vi "Programa_da_Aplicação_Hold_UP.vi"() -> ()   [LabVIEW 2019]
uses:
  Variaveis_Globais_CLP_Paralelo.vi
panel:
  in  "SPW-INV-001":bool
  in  "SPK-INV-001":bool
  in  "Condição_Hold_up_Vini":bool
  in  "Valores_Instrumentos":T1 {"DeltaP_K" format="%#_6e"; "DeltaP_W" format="%#_6e"; "Diâmetro Tubulação [m]" format="%#_6e"; "PC-TQ-TD" format="%#_6e"; "PC-TQ-TI" format="%#_6e"; "PC-TQ-GP" format="%#_6e"; "PC-TQ-PV" format="%#_6e"; "PC-TQ-SP" format="%#_6e"; "PC-TQ-OV" format="%#_6e"; "SPW-WR-VEL" format="%#_6e"; "SPK-WR-VEL" format="%#_6e"; "SKM-PC-TQ" format="%#_6e"; "SKM-FC-KF" format="%#_6e"; "SKM-FC-WF" format="%#_6e"; "SKM-FC-AR" format="%#_6e"; "SKM-TI-KF_COR" format="%#_6e"; "SKS-LC-K" format="%#_6e"; "SPK-RD-CRT" format="%#_6e"; "SPW-RD-CRT" format="%#_6e"; "SKM-FIC-AR_COR" format="%#_6e"; "SKM-FIC-KF_COR" format="%#_6e"; "SKM-AI-AR_COR" format="%#_6e"; "SKM-AI-KF_COR" format="%#_6e"; "SKM-TI-AR_COR" format="%#_6e"; "SKM-TI-KF" format="%#_6e"; "SPW-RD-VEL" format="%#_6e"; "SPK-RD-VEL" format="%#_6e"; "SKS-LC-W" format="%#_6e"; "SIT-PI-002" format="%#_6e"; "SKM-FI-WF" format="%#_6e"; "SKM-TI-WF" format="%#_6e"; "SKM-PI-BAR" format="%#_6e"; "SKM-PI-LAM" format="%#_6e"; "SMA-PI-LAM" format="%#_6e"; "SMA-TI-LAM" format="%#_6e"; "SKM-PI-TQ" format="%#_6e"; "SKM-TI-TQ" format="%#_6e"}
  in  "stop":bool
  in  "SPK-WR-VEL":dbl caption="SPK-WR-VEL [%]"
  in  "SPW-WR-VEL":dbl caption="SPW-WR-VEL [%]"
  in  "SKM-FC-TQ":dbl caption="SKM-FC-TQ [%]"
  in  "SKM-FC-AR":dbl caption="SKM-FC-AR [%]"
  in  "SKM-FC-WF":dbl caption="SKM-FC-WF [%]"
  in  "SKM-FC-KF":dbl caption="SKM-FC-KF [%]"
  in  "Variaveis_Aplicações":T2
  # "Controle de Valvulas"
  # "Controle de Bombas"
  # "Espaço Delimitado para criação do Painel Frontal \nque será utilizado nessa aplicação."
  # "SKID MEDI敲O - LEITURA"
  # "SKID MEDI敲O - ESCRITA"
  # "SKID BOMBA - ESCRITA"
  # "SKID BOMBA - LEITURA"
  # "SKID SEPARA敲O - LEITURA"
  # "SKID INJE敲O - LEITURA"
  # "SKID BOMBA"
  # "SKID DE MEDI敲O"
  # "SKID DE SEPARA敲O"
  # "SKID DE INJE敲O"
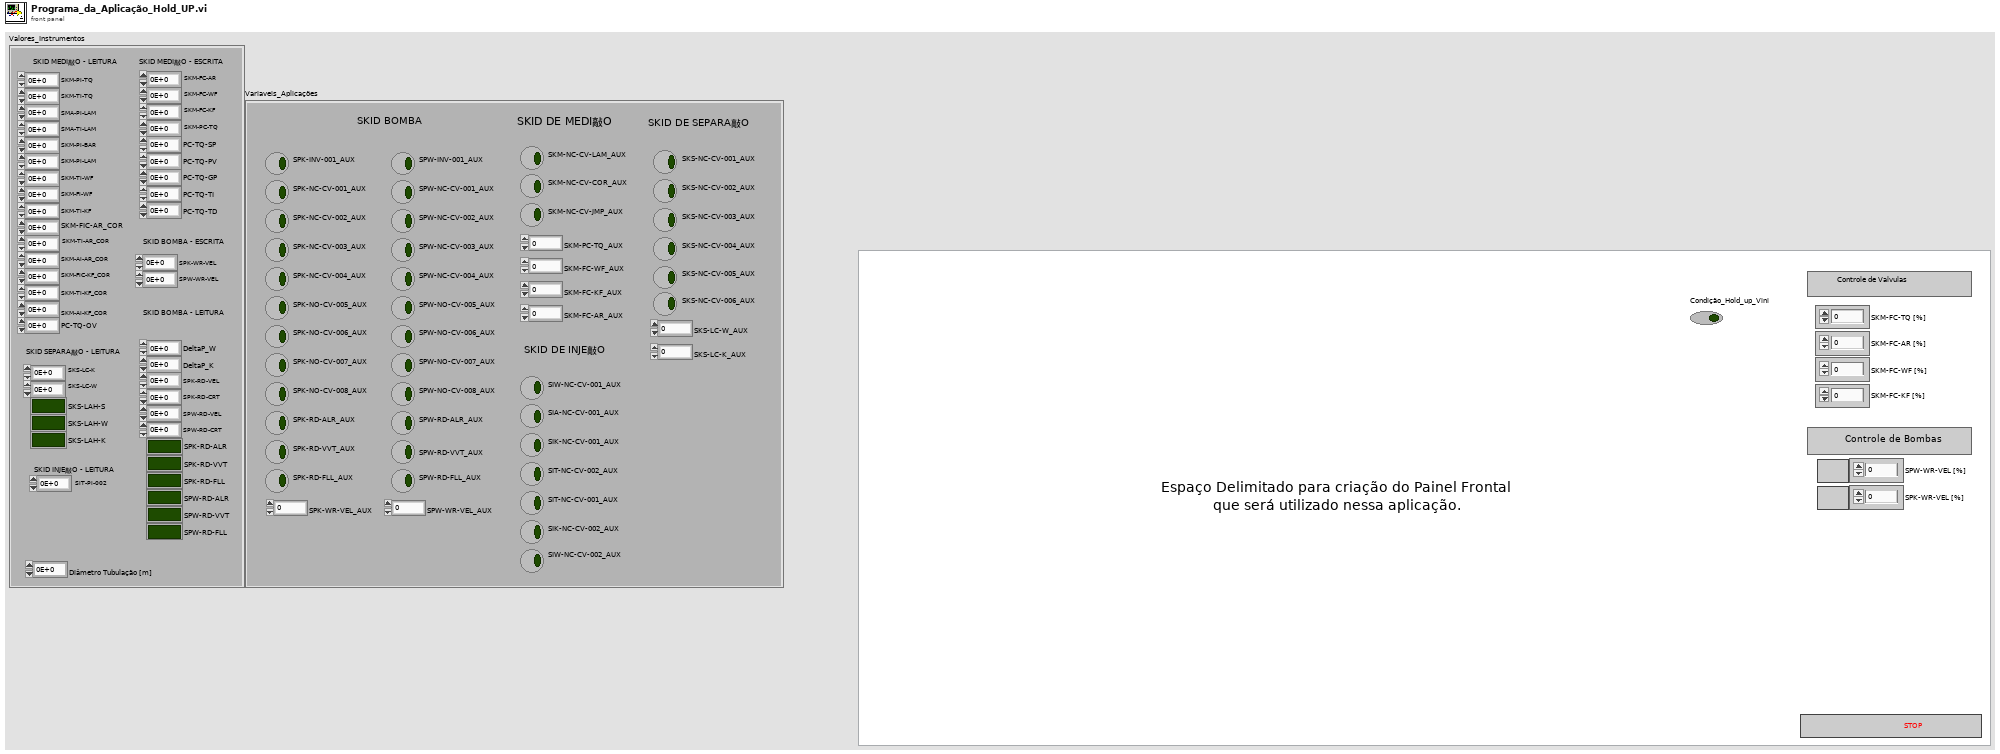
[diagram p1: front panel]
types:
  T1 = cluster{"SKM-TI-TQ":dbl, "SKM-PI-TQ":dbl, "SMA-TI-LAM":dbl, "SMA-PI-LAM":dbl, "SKM-PI-LAM":dbl, "SKM-PI-BAR":dbl, "SKM-TI-WF":dbl, "SKM-FI-WF":dbl, "SIT-PI-002":dbl, "SKS-LC-W":dbl, "SPK-RD-VEL":dbl, "SPW-RD-VEL":dbl, "SKM-TI-KF":dbl, "SKM-TI-AR_COR":dbl, "SKM-AI-KF_COR":dbl, "SKM-AI-AR_COR":dbl, "SKM-FIC-KF_COR":dbl, "SKM-FIC-AR_COR":dbl, "SPW-RD-CRT":dbl, "SPK-RD-CRT":dbl, "SKS-LC-K":dbl, "SKM-TI-KF_COR":dbl, "SKM-FC-AR":dbl, "SKM-FC-WF":dbl, "SKM-FC-KF":dbl, "SKM-PC-TQ":dbl, "SPK-WR-VEL":dbl, "SPW-WR-VEL":dbl, "SPK-RD-ALR":bool, "SPK-RD-VVT":bool, "SPK-RD-FLL":bool, "SPW-RD-ALR":bool, "SPW-RD-VVT":bool, "SPW-RD-FLL":bool, "PC-TQ-OV":dbl, "PC-TQ-SP":dbl, "PC-TQ-PV":dbl, "PC-TQ-GP":dbl, "PC-TQ-TI":dbl, "PC-TQ-TD":dbl, "SKS-LAH-S":bool, "SKS-LAH-W":bool, "SKS-LAH-K":bool, "Diâmetro Tubulação [m]":dbl, "DeltaP_W":dbl, "DeltaP_K":dbl}
  T2 = cluster{"SPK-NC-CV-001_AUX":bool, "SPK-NC-CV-002_AUX":bool, "SPK-NC-CV-003_AUX":bool, "SPK-NC-CV-004_AUX":bool, "SPK-NO-CV-005_AUX":bool, "SPK-NO-CV-006_AUX":bool, "SPK-NO-CV-007_AUX":bool, "SPK-NO-CV-008_AUX":bool, "SIW-NC-CV-001_AUX":bool, "SIA-NC-CV-001_AUX":bool, "SIK-NC-CV-001_AUX":bool, "SIT-NC-CV-002_AUX":bool, "SIT-NC-CV-001_AUX":bool, "SIK-NC-CV-002_AUX":bool, "SIW-NC-CV-002_AUX":bool, "SKS-NC-CV-001_AUX":bool, "SKS-NC-CV-002_AUX":bool, "SKS-NC-CV-003_AUX":bool, "SPK-INV-001_AUX":bool, "SPW-NC-CV-001_AUX":bool, "SPW-NC-CV-002_AUX":bool, "SPW-NC-CV-003_AUX":bool, "SPW-NC-CV-004_AUX":bool, "SPW-NO-CV-005_AUX":bool, "SPW-NO-CV-006_AUX":bool, "SPW-NO-CV-007_AUX":bool, "SPW-NO-CV-008_AUX":bool, "SPW-INV-001_AUX":bool, "SKM-NC-CV-LAM_AUX":bool, "SKM-NC-CV-COR_AUX":bool, "SKM-NC-CV-JMP_AUX":bool, "SKM-FC-AR_AUX":dbl, "SPK-RD-ALR_AUX":bool, "SPK-RD-VVT_AUX":bool, "SPK-RD-FLL_AUX":bool, "SPK-WR-VEL_AUX":dbl, "SPW-RD-ALR_AUX":bool, "SPW-RD-VVT_AUX ":bool, "SPW-RD-FLL_AUX ":bool, "SPW-WR-VEL_AUX ":dbl, "SKS-NC-CV-004_AUX":bool, "SKS-NC-CV-005_AUX":bool, "SKS-LC-W_AUX":dbl, "SKS-LC-K_AUX":dbl, "SKM-PC-TQ_AUX":dbl, "SKM-FC-WF_AUX":dbl, "SKM-FC-KF_AUX":dbl, "SKS-NC-CV-006_AUX":bool}
  T3 = enum8{"Enabled", "Disabled", "Disabled and Grayed Out"}
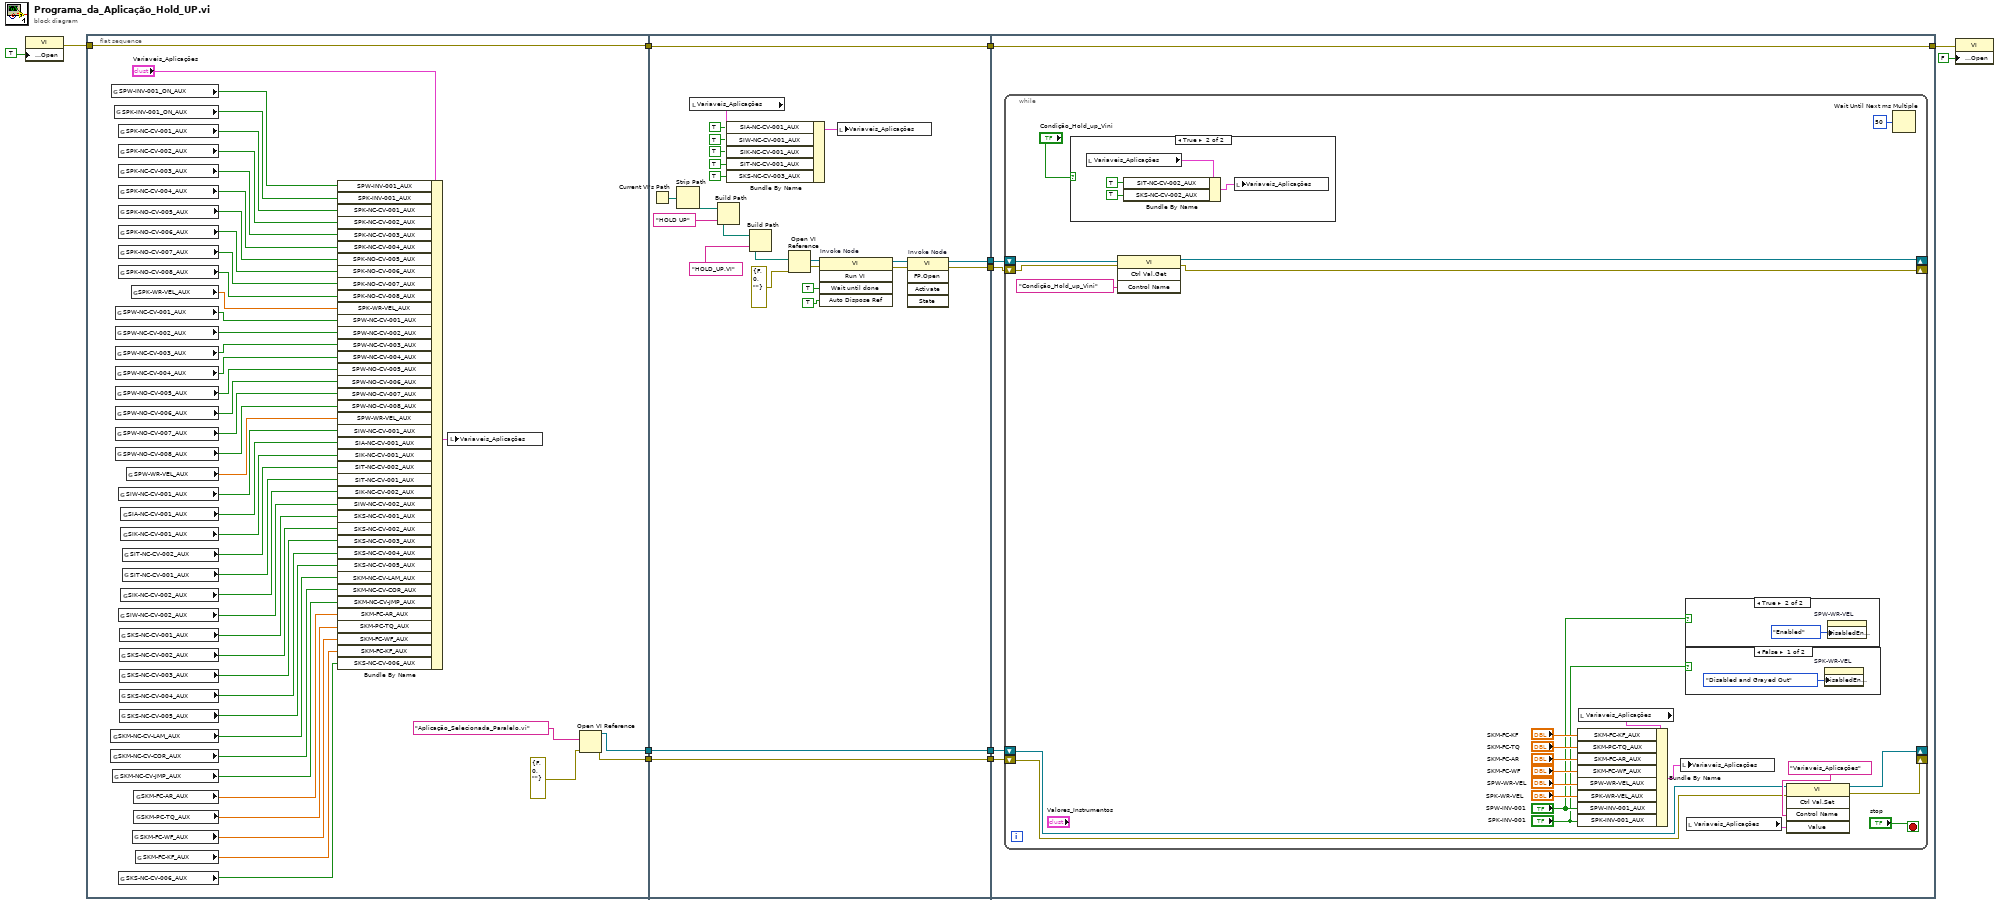
[diagram p0: block diagram]
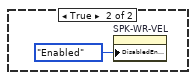
[diagram p2: hidden frame]
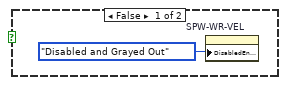
[diagram p3: hidden frame]
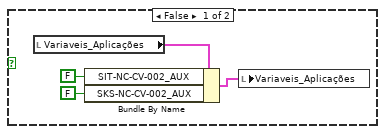
[diagram p4: hidden frame]
diagram:
  n1 = property class="VI"("Front Panel.Open"=TRUE ("Front Panel Window:Open")) -> (error out=w11:errorcluster)  [unwired: 2 in, 1 out]
  n2 = flat-sequence {
    tunnel: [w21] -> w8
    tunnel: w11 -> [w21]
    tunnel: [w19] -> w6
    tunnel: [w18] -> w4
    tunnel: w8 -> [w84]
    tunnel: [w84] -> w7
    tunnel: w6 -> [w83]
    tunnel: [w83] -> w5
    tunnel: w4 -> [w82]
    tunnel: [w82] -> w3
    tunnel: [w61] -> w2
    tunnel: [w60] -> w1
    tunnel: w7 -> [w89]
    tunnel: [w89] -> w12
    tunnel: w5 -> [w88]
    tunnel: w3 -> [w87]
    tunnel: w2 -> [w86]
    tunnel: w1 -> [w85]
    frame #0 {
      n3 = global read "Variaveis_Globais_CLP_Paralelo.vi" "SKM-NC-CV-LAM_AUX"() -> (w53:bool)
      n4 = global read "Variaveis_Globais_CLP_Paralelo.vi" "SKM-NC-CV-COR_AUX"() -> (w54:bool)
      n5 = global read "Variaveis_Globais_CLP_Paralelo.vi" "SPW-INV-001_ON_AUX"() -> (w14:bool)
      n6 = global read "Variaveis_Globais_CLP_Paralelo.vi" "SKM-NC-CV-JMP_AUX"() -> (w55:bool)
      n7 = global read "Variaveis_Globais_CLP_Paralelo.vi" "SPK-INV-001_ON_AUX"() -> (w13:bool)
      n8 = global read "Variaveis_Globais_CLP_Paralelo.vi" "SPW-NC-CV-001_AUX"() -> (w32:bool)
      n9 = global read "Variaveis_Globais_CLP_Paralelo.vi" "SPW-NC-CV-002_AUX"() -> (w31:bool)
      n10 = global read "Variaveis_Globais_CLP_Paralelo.vi" "SPW-NC-CV-003_AUX"() -> (w30:bool)
      n11 = global read "Variaveis_Globais_CLP_Paralelo.vi" "SPW-NC-CV-004_AUX"() -> (w29:bool)
      n12 = global read "Variaveis_Globais_CLP_Paralelo.vi" "SPW-NO-CV-005_AUX"() -> (w28:bool)
      n13 = global read "Variaveis_Globais_CLP_Paralelo.vi" "SPW-NO-CV-006_AUX"() -> (w27:bool)
      n14 = global read "Variaveis_Globais_CLP_Paralelo.vi" "SPW-NO-CV-007_AUX"() -> (w26:bool)
      n15 = global read "Variaveis_Globais_CLP_Paralelo.vi" "SPW-NO-CV-008_AUX"() -> (w25:bool)
      n16 = global read "Variaveis_Globais_CLP_Paralelo.vi" "SPK-NC-CV-001_AUX"() -> (w23:bool)
      n17 = global read "Variaveis_Globais_CLP_Paralelo.vi" "SPK-NC-CV-002_AUX"() -> (w40:bool)
      n18 = global read "Variaveis_Globais_CLP_Paralelo.vi" "SPK-NC-CV-003_AUX"() -> (w39:bool)
      n19 = global read "Variaveis_Globais_CLP_Paralelo.vi" "SPK-NC-CV-004_AUX"() -> (w38:bool)
      n20 = global read "Variaveis_Globais_CLP_Paralelo.vi" "SPK-NO-CV-005_AUX"() -> (w37:bool)
      n21 = global read "Variaveis_Globais_CLP_Paralelo.vi" "SPK-NO-CV-006_AUX"() -> (w36:bool)
      n22 = global read "Variaveis_Globais_CLP_Paralelo.vi" "SPK-NO-CV-007_AUX"() -> (w35:bool)
      n23 = global read "Variaveis_Globais_CLP_Paralelo.vi" "SPK-NO-CV-008_AUX"() -> (w34:bool)
      n24 = global read "Variaveis_Globais_CLP_Paralelo.vi" "SIW-NC-CV-001_AUX"() -> (w41:bool)
      n25 = global read "Variaveis_Globais_CLP_Paralelo.vi" "SIW-NC-CV-002_AUX"() -> (w47:bool)
      n26 = global read "Variaveis_Globais_CLP_Paralelo.vi" "SKS-NC-CV-006_AUX"() -> (w15:bool)
      n27 = global read "Variaveis_Globais_CLP_Paralelo.vi" "SKS-NC-CV-001_AUX"() -> (w48:bool)
      n28 = global read "Variaveis_Globais_CLP_Paralelo.vi" "SKS-NC-CV-002_AUX"() -> (w49:bool)
      n29 = global read "Variaveis_Globais_CLP_Paralelo.vi" "SKS-NC-CV-003_AUX"() -> (w50:bool)
      n30 = global read "Variaveis_Globais_CLP_Paralelo.vi" "SKS-NC-CV-004_AUX"() -> (w51:bool)
      n31 = global read "Variaveis_Globais_CLP_Paralelo.vi" "SKS-NC-CV-005_AUX"() -> (w52:bool)
      n32 = global read "Variaveis_Globais_CLP_Paralelo.vi" "SIA-NC-CV-001_AUX"() -> (w42:bool)
      n33 = global read "Variaveis_Globais_CLP_Paralelo.vi" "SIK-NC-CV-001_AUX"() -> (w43:bool)
      n34 = global read "Variaveis_Globais_CLP_Paralelo.vi" "SIK-NC-CV-002_AUX"() -> (w46:bool)
      n35 = global read "Variaveis_Globais_CLP_Paralelo.vi" "SIT-NC-CV-002_AUX"() -> (w44:bool)
      n36 = global read "Variaveis_Globais_CLP_Paralelo.vi" "SIT-NC-CV-001_AUX"() -> (w45:bool)
      n37 = global read "Variaveis_Globais_CLP_Paralelo.vi" "SPW-WR-VEL_AUX"() -> (w24:dbl)
      n38 = global read "Variaveis_Globais_CLP_Paralelo.vi" "SPK-WR-VEL_AUX"() -> (w33:dbl)
      n39 = global read "Variaveis_Globais_CLP_Paralelo.vi" "SKM-FC-WF_AUX"() -> (w58:dbl)
      n40 = global read "Variaveis_Globais_CLP_Paralelo.vi" "SKM-FC-AR_AUX"() -> (w56:dbl)
      n41 = global read "Variaveis_Globais_CLP_Paralelo.vi" "SKM-PC-TQ_AUX"() -> (w57:dbl)
      n42 = global read "Variaveis_Globais_CLP_Paralelo.vi" "SKM-FC-KF_AUX"() -> (w59:dbl)
      n43 = Bundle By Name(cluster="Variaveis_Aplicações", "SPW-INV-001_AUX"=w14, "SPK-INV-001_AUX"=w13, "SPK-NC-CV-001_AUX"=w23, "SPK-NC-CV-002_AUX"=w40, "SPK-NC-CV-003_AUX"=w39, "SPK-NC-CV-004_AUX"=w38, "SPK-NO-CV-005_AUX"=w37, "SPK-NO-CV-006_AUX"=w36, "SPK-NO-CV-007_AUX"=w35, "SPK-NO-CV-008_AUX"=w34, "SPK-WR-VEL_AUX"=w33, "SPW-NC-CV-001_AUX"=w32, "SPW-NC-CV-002_AUX"=w31, "SPW-NC-CV-003_AUX"=w30, "SPW-NC-CV-004_AUX"=w29, "SPW-NO-CV-005_AUX"=w28, "SPW-NO-CV-006_AUX"=w27, "SPW-NO-CV-007_AUX"=w26, "SPW-NO-CV-008_AUX"=w25, "SPW-WR-VEL_AUX"=w24, "SIW-NC-CV-001_AUX"=w41, "SIA-NC-CV-001_AUX"=w42, "SIK-NC-CV-001_AUX"=w43, "SIT-NC-CV-002_AUX"=w44, "SIT-NC-CV-001_AUX"=w45, "SIK-NC-CV-002_AUX"=w46, "SIW-NC-CV-002_AUX"=w47, "SKS-NC-CV-001_AUX"=w48, "SKS-NC-CV-002_AUX"=w49, "SKS-NC-CV-003_AUX"=w50, "SKS-NC-CV-004_AUX"=w51, "SKS-NC-CV-005_AUX"=w52, "SKM-NC-CV-LAM_AUX"=w53, "SKM-NC-CV-COR_AUX"=w54, "SKM-NC-CV-JMP_AUX"=w55, "SKM-FC-AR_AUX"=w56, "SKM-PC-TQ_AUX"=w57, "SKM-FC-WF_AUX"=w58, "SKM-FC-KF_AUX"=w59, "SKS-NC-CV-006_AUX"=w15) -> (w22:T2)
      n44 = local write "Variaveis_Aplicações"(w22) -> ()
      n45 = Open VI Reference(vi path="Aplicação_Selecionada_Paralelo.vi" ("y"), error in (no error)=errorcluster {"status"=FALSE, "code"=0, "source"=""}) -> (vi reference=w19:refnum<vi>, error out=w18:errorcluster)  [unwired: 4 in]
    }
    frame #1 {
      n46 = Current VI's Path() -> (path=w62:path)
      n47 = Strip Path(path=w62) -> (stripped path=w63:path)  [unwired: 1 out]
      n48 = local read "Variaveis_Aplicações"() -> (w81:T2)
      n49 = Build Path(base path=w63, name or relative path="HOLD UP") -> (appended path=w65:path)
      n50 = Bundle By Name(cluster=w81, "SIA-NC-CV-001_AUX"=TRUE, "SIW-NC-CV-001_AUX"=TRUE, "SIK-NC-CV-001_AUX"=TRUE, "SIT-NC-CV-001_AUX"=TRUE, "SKS-NC-CV-003_AUX"=TRUE) -> (w80:T2)
      n51 = Build Path(base path=w65, name or relative path="HOLD_UP.VI") -> (appended path=w68:path)
      n52 = Open VI Reference(vi path=w68, error in (no error)=errorcluster {"status"=FALSE, "code"=0, "source"=""}) -> (vi reference=w73:refnum<vi>, error out=w74:errorcluster)  [unwired: 4 in]
      n53 = invoke on="Invoke Node" class="VI" method="Run VI"(reference=w73, error in=w74, "Wait until done"=TRUE ("Wait Until Done"), "Auto Dispose Ref"=TRUE ("Auto Dispose Reference")) -> (reference out=w71:refnum<vi>, error out=w72:errorcluster)  [unwired: 1 in, 3 out]
      n54 = local write "Variaveis_Aplicações"(w80) -> ()
      n55 = invoke on="Invoke Node" class="VI" method="FP.Open"(reference=w71, error in=w72) -> (reference out=w61:refnum<vi>, error out=w60:errorcluster)  [unwired: 3 in, 3 out]
    }
    frame #2 {
      n56 = while {
        shift-right: [w109] -> _
        shift-left: w88 -> [w110]
        shift-right: [w108] -> _
        shift-left: w87 -> [w107]
        shift-right: [w94] -> _
        shift-left: w86 -> [w96]
        shift-right: [w93] -> _
        shift-left: w85 -> [w95]
        stop <- "stop" stop-if-true
        n57 = case shown="True" "Condição_Hold_up_Vini" {
          frame False {
            n58 = local read "Variaveis_Aplicações"() -> (w118:T2)
            n59 = Bundle By Name(cluster=w118, "SIT-NC-CV-002_AUX"=FALSE, "SKS-NC-CV-002_AUX"=FALSE) -> (w119:T2)
            n60 = local write "Variaveis_Aplicações"(w119) -> ()
          }
          frame True {
            n61 = local read "Variaveis_Aplicações"() -> (w122:T2)
            n62 = Bundle By Name(cluster=w122, "SIT-NC-CV-002_AUX"=TRUE, "SKS-NC-CV-002_AUX"=TRUE) -> (w123:T2)
            n63 = local write "Variaveis_Aplicações"(w123) -> ()
          }
        }
        n64 = invoke class="VI" method="Ctrl Val.Get"(reference=w96, error in=w95, "Control Name"="Condição_Hold_up_Vini") -> (reference out=w94:refnum<vi>, error out=w93:errorcluster)  [unwired: 1 in, 2 out]
        n65 = local read "Variaveis_Aplicações"() -> (w106:T2)
        n66 = Bundle By Name(cluster=w106, "SKM-FC-KF_AUX"="SKM-FC-KF", "SKM-PC-TQ_AUX"="SKM-FC-TQ", "SKM-FC-AR_AUX"="SKM-FC-AR", "SKM-FC-WF_AUX"="SKM-FC-WF", "SPW-WR-VEL_AUX"="SPW-WR-VEL", "SPK-WR-VEL_AUX"="SPK-WR-VEL", "SPW-INV-001_AUX"="SPW-INV-001", "SPK-INV-001_AUX"="SPK-INV-001") -> (w105:T2)
        n67 = local write "Variaveis_Aplicações"(w105) -> ()
        n68 = case shown="True" "SPW-INV-001" {
          frame False {
            n69 = property on="SPW-WR-VEL" class="DigNum (strict)"("DisabledEnum"=T3."Disabled and Grayed Out" ("Disabled")) -> ()  [unwired: 2 in, 2 out]
          }
          frame True {
            n70 = property on="SPW-WR-VEL" class="DigNum (strict)"("DisabledEnum"=T3."Enabled" ("Disabled")) -> ()  [unwired: 2 in, 2 out]
          }
        }
        n71 = case shown="False" "SPK-INV-001" {
          frame False {
            n72 = property on="SPK-WR-VEL" class="DigNum (strict)"("DisabledEnum"=T3."Disabled and Grayed Out" ("Disabled")) -> ()  [unwired: 2 in, 2 out]
          }
          frame True {
            n73 = property on="SPK-WR-VEL" class="DigNum (strict)"("DisabledEnum"=T3."Enabled" ("Disabled")) -> ()  [unwired: 2 in, 2 out]
          }
        }
        n74 = local read "Variaveis_Aplicações"() -> (w111:T2)
        n75 = invoke class="VI" method="Ctrl Val.Set"(reference=w110, error in=w107, "Control Name"="Variaveis_Aplicações", "Value"=w111) -> (reference out=w109:refnum<vi>, error out=w108:errorcluster)  [unwired: 1 in, 3 out]
        n76 = Wait Until Next ms Multiple(millisecond multiple=u32 50) -> ()  [unwired: 1 out]
      }
    }
  }
  n77 = property class="VI"(error in=w12, "Front Panel.Open"=FALSE ("Front Panel Window:Open")) -> ()  [unwired: 1 in, 2 out]
